vi "Set Brower View .vi"(8 "error in (no error)":errorcluster, 10 "Brower View.lvclass":refnum<class "Brower View.lvclass">, 11 "Browers in":refnum<class "Browers Controller.lvclass">) -> (0 "error out":errorcluster, 3 "Browers out":refnum<class "Browers Controller.lvclass">)   [LabVIEW 2015, in "Browers Controller.lvclass"]
uses:
  Browers Controller.lvclass
  Brower View/Brower View.lvclass
  Browers Controller.lvclass/Browers Controller.ctl
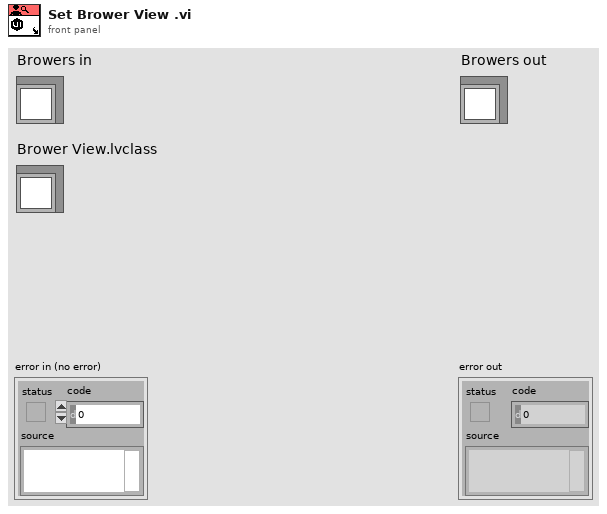
[diagram p1: front panel]
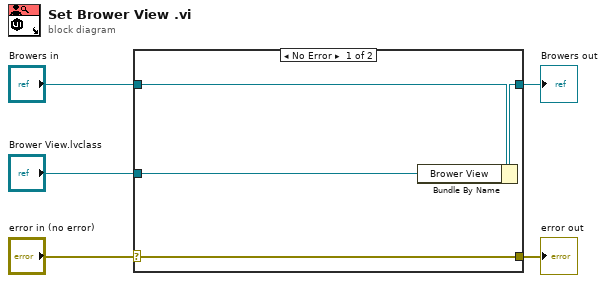
[diagram p0: block diagram]
diagram:
  n1 = case shown="No Error" "error in (no error)" {
    selector: "error in (no error)" -> [w9 w10]
    tunnel: [w9 w10] -> w4
    tunnel: [w7 w11] -> w2
    tunnel: "Browers in" -> [w8 w11]
    tunnel: "Brower View.lvclass" -> [w6 _]
    frame No Error {
      n2 = Bundle By Name(cluster=w8, "Brower View"=w6) -> (w7:refnum<class "Browers Controller.lvclass">)
    }
    frame Error {
    }
  }
  "error out" <- w4
  "Browers out" <- w2
